vi "GeneradorFunciones.vi"() -> ()   [LabVIEW 2016]
panel:
  in  "BOOL1":bool
  in  "Frecuencia":u32
  in  "Offset":dbl(knob) scale=-10.0..10.0
  in  "Amplitud":dbl(knob) scale=-10.0..10.0
  in  "DC":dbl(knob) scale=0.0..10.0
  out "Waveform Chart":dbl(graph)
  in  "Enum":T1(ring)
  out "Numeric Indicator":dbl
  in  "Stop Button":bool
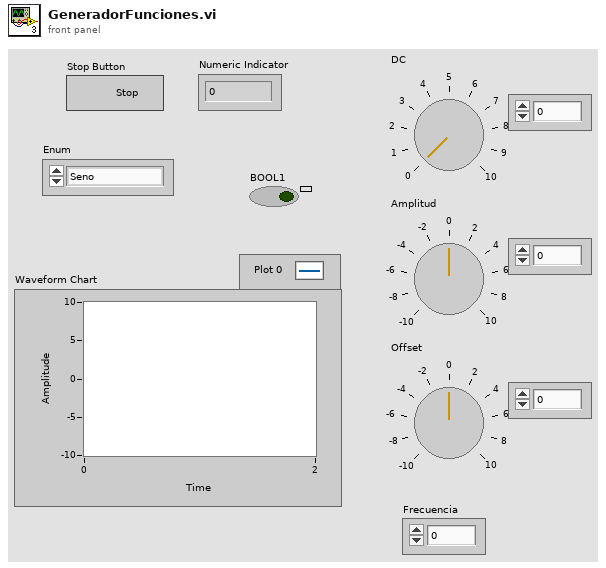
[diagram p1: front panel]
types:
  T1 = enum16{"Seno", "Triangular", "Diente de sierra", "Pulso", "Secante", "DC", "GND", "SAMPLING", "COSECANTE", "TANGENTE", "COTANGENTE", "COSENO"}
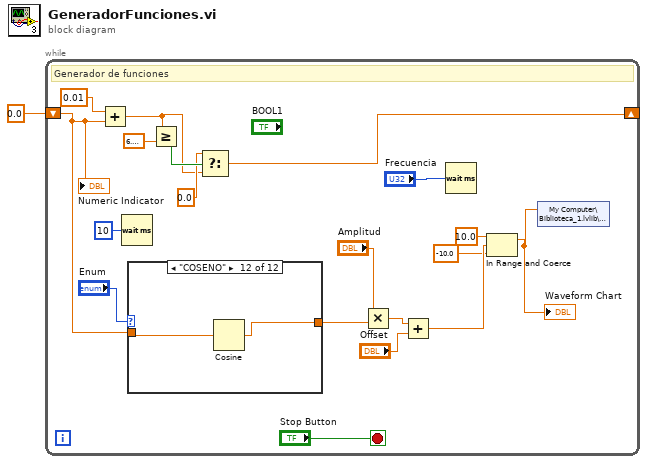
[diagram p0: block diagram]
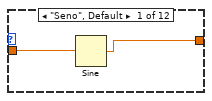
[diagram p2: hidden frame]
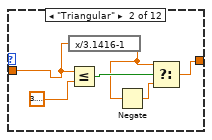
[diagram p3: hidden frame]
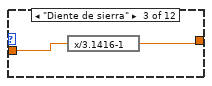
[diagram p4: hidden frame]
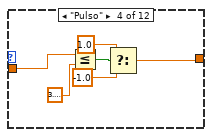
[diagram p5: hidden frame]
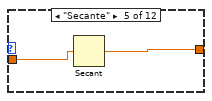
[diagram p6: hidden frame]
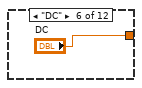
[diagram p7: hidden frame]
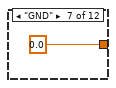
[diagram p8: hidden frame]
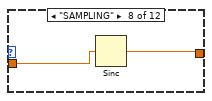
[diagram p9: hidden frame]
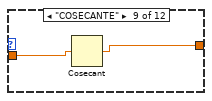
[diagram p10: hidden frame]
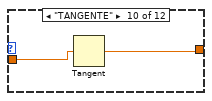
[diagram p11: hidden frame]
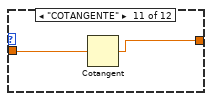
[diagram p12: hidden frame]
diagram:
  n1 = while {
    shift-right: [w13] -> _
    shift-left: 0.0 -> [w11]
    stop <- "Stop Button" stop-if-true
    # "Generador de funciones"
    n2 = Add(x=0.01, y=w11) -> (x+y=w14:dbl)
    n3 = Wait (ms)(milliseconds to wait=u32 10) -> ()  [unwired: 1 out]
    n4 = case shown="\"COSENO\"" "Enum" {
      tunnel: w11 -> [w22 w26 w30 w36 w38 _ _ w42 w44 w46 w48 w50]
      tunnel: [w21 w25 w29 w31 w37 "DC" 0.0 ("f") w41 w43 w45 w47 w49] -> w10
      frame "Seno", Default {
        n5 = Sine(x=w22) -> (sin(x)=w21:dbl)
      }
      frame "Triangular" {
        n6 = expression code="x/3.1416-1"(w26) -> (w23:dbl)
        n7 = Less Or Equal?(x=w26, y=3.141592653589793) -> (x <= y?=w27:bool)
        n8 = Negate(x=w23) -> (-x=w24:dbl)
        n9 = Select(t=w23, s=w27, f=w24) -> (s? t:f=w25:dbl)
      }
      frame "Diente de sierra" {
        n10 = expression code="x/3.1416-1"(w30) -> (w29:dbl)
      }
      frame "Pulso" {
        n11 = Less Or Equal?(x=w36, y=3.141592653589793) -> (x <= y?=w34:bool)
        n12 = Select(t=1.0, s=w34, f=-1.0) -> (s? t:f=w31:dbl)
      }
      frame "Secante" {
        n13 = Secant(1:w38) -> (0:w37:dbl)
      }
      frame "DC" {
      }
      frame "GND" {
      }
      frame "SAMPLING" {
        n14 = Sinc(1:w42) -> (0:w41:dbl)
      }
      frame "COSECANTE" {
        n15 = Cosecant(1:w44) -> (0:w43:dbl)
      }
      frame "TANGENTE" {
        n16 = Tangent(1:w46) -> (0:w45:dbl)
      }
      frame "COTANGENTE" {
        n17 = Cotangent(1:w48) -> (0:w47:dbl)
      }
      frame "COSENO" {
        n18 = Cosine(x=w50) -> (cos(x)=w49:dbl)
      }
    }
    n19 = Greater Or Equal?(x=w14, y=6.283185307179586) -> (x >= y?=w16:bool)
    n20 = Select(t=0.0, s=w16, f=w14) -> (s? t:f=w13:dbl)
    n21 = Multiply(x="Amplitud", y=w10) -> (x*y=w8:dbl)
    n22 = Add(x=w8, y="Offset") -> (x+y=w5:dbl)
    n23 = Wait (ms)(milliseconds to wait="Frecuencia") -> ()  [unwired: 1 out]
    n24 = In Range and Coerce(upper limit=10.0, x=w5, lower limit=-10.0) -> (coerced(x)=w2:dbl)  [unwired: 1 out]
    "Waveform Chart" <- w2
    n25 = shared-variable "My Computer\\Biblioteca_1.lvlib\\DBL1"(w2) -> ()  [unwired: 1 in, 1 out]
    "Numeric Indicator" <- w11
  }
